vi "GetSystemHWInfo.vi"(8 "error in (no error)":errorcluster) -> (0 "error out":errorcluster, 3 "system info":T1, 5 "Found?":bool)   [LabVIEW 2017, in "SystemInfoProcess.lvlib"]
doc: "Gets information about system hardware."
uses:
  <vilib>/addons/SystemInfoProcess/SystemInfoProcess.lvlib
  <vilib>/addons/cRIODetectHW/control/SystemHW.ctl
  <vilib>/addons/cRIODetectHW/control/cRIO Product Info.ctl
  <vilib>/addons/PointValueMap/subVIs/Point_Read_variant.vi
  <vilib>/addons/PointValueMap/PointValueMap.lvlib
  <vilib>/addons/cRIODetectHW/cRIODetectHW.lvlib
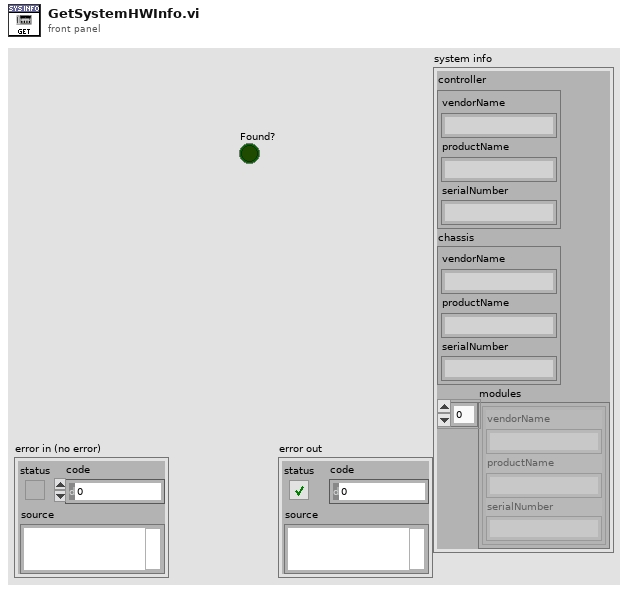
[diagram p1: front panel]
types:
  T1 = typedef "cRIODetectHW.lvlib/SystemHW.ctl" = cluster{"controller":T2, "chassis":T2, "modules":T2[]}
  T2 = typedef "cRIODetectHW.lvlib/cRIO Product Info.ctl" = cluster{"vendorName":string, "productName":string, "serialNumber":string}
  T3 = typedef "PointValueMap.lvlib/PointMap.ctl" = refnum<data-value>
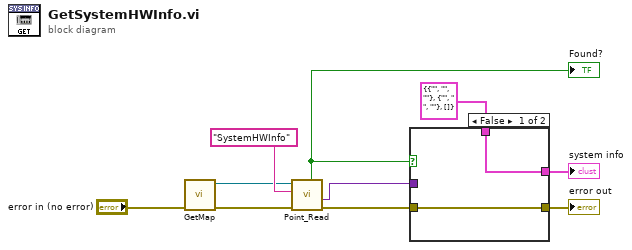
[diagram p0: block diagram]
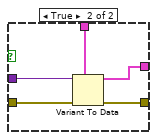
[diagram p2: hidden frame]
diagram:
  n1 = call <vilib>:"GetMap.vi"("error in (no error)"="error in (no error)") -> ("error out"=w5:errorcluster, "SystemInfoMap"=w4:T3)  [unwired: 9 in]
  n2 = call-poly <vilib>:"Point_Read.vi"("Error In"=w5, "Tag"="SystemHWInfo", "Map"=w4) -> ("Error Out"=w10:errorcluster, "Value"=w7:variant, "Valid?"=w6:bool)  [unwired: 3 in, 3 out]
  "Found?" <- w6
  n3 = case shown="False" w6 {
    tunnel: w10 -> [w11 w17]
    tunnel: [w11 w16] -> w9
    tunnel: T1 {"controller"={"vendorName"="", "productName"="", "serialNumber"=""}, "chassis"={"vendorName"="", "productName"=" ", "serialNumber"=""}, "modules"=[]} ("system info") -> [w12 w15]
    tunnel: [w12 w14] -> w1
    tunnel: w7 -> [_ w13]
    frame False {
    }
    frame True {
      n4 = Variant To Data(error in=w17, type=w15, Variant=w13) -> (data=w14:T1, error out=w16:errorcluster)
    }
  }
  "error out" <- w9
  "system info" <- w1
